vi "Dashboard Main.vi"() -> ()   [LabVIEW 2014]
uses:
  <vilib>/event_ctls.llb/eventvkey.ctl
  <vilib>/Rock Robotics/WPI/Dashboard/WPI_DashboardLogging Global.vi
  <vilib>/Utility/config.llb/Write Key (String).vi
  <vilib>/Utility/config.llb/Write Key (I32).vi
  <vilib>/Utility/config.llb/NI_LVConfig.lvlib
panel:
  in  "TCP":refnum<k5>
  in  "Rec Mode":enum32{"Stop", "Record", "Playback"}(radio)
  in  "Vision":u16(ring) items=["Camera Off", "USB Camera SW", "USB Camera HW", "IP Camera"]
  out "Camera IP":string
  out "Image Message":string="Timeout in Camera Communications"
  in  "Dashboard Tab":T1(tab)
  in  "Camera Settings":T2={"Frame Rate"=30, "Compression"=30, "Size"=1} {"Frame Rate" scale=1.0..30.0; "Size" items=["640x480", "320x240", "160x120"]}
  out "MotorChart R":cluster{"Numeric":dbl, "Numeric":dbl}(graph)
  out "MotorChart L":T3(graph)
  out "MotorSliders R":cluster{"MotorSlide1":dbl, "MotorSlide2":dbl} {"MotorSlide2" scale=-1.0..1.0 scale format="%#_2e"; "MotorSlide1" scale=-1.0..1.0 scale format="%#_2e"}
  out "MotorSliders L":T4 {"MotorSlide4 2" scale=0.0..14.0 scale format="%#_2e"; "MotorSlide2" scale=-1.0..1.0 scale format="%#_2e"; "MotorSlide1" scale=-1.0..1.0 scale format="%#_2e"}
  out "JS1 Z":dbl(slide) scale=-1.0..1.0 scale format="%#_2e"
  out "JS1 Graph":cluster{"X":dbl, "Y":dbl}[](graph)
  out "JS1 Buttons":T5
  out "JS2 Z":dbl(slide) scale=-1.0..1.0 scale format="%#_2e"
  out "JS2 Graph":cluster{"X":dbl, "Y":dbl}[](graph)
  out "JS2 Buttons":T5
  out "Mode":T6(ring)=enum."Auto Disabled"
  in  "DB Camera Config":bool
  out "fps":dbl format="%#.1g"
  out "Mbps":dbl format="%#.1g"
  out "Mbps 2":bool
  in  "DB/String 9":string
  in  "DB/String 8":string
  in  "DB/String 7":string
  in  "DB/String 6":string
  in  "DB/String 5":string
  in  "DB/String 4":string
  in  "DB/String 3":string
  in  "DB/String 2":string
  in  "DB/String 1":string
  in  "DB/String 0":string
  in  "DB/Slider 0":dbl(slide) scale=0.0..5.0
  in  "DB/Slider 1":dbl(slide) scale=0.0..5.0
  in  "DB/Slider 2":dbl(slide) scale=0.0..5.0
  in  "DB/Slider 3":dbl(slide) scale=0.0..5.0
  out "DB/LED 3":bool
  out "DB/LED 2":bool
  out "DB/LED 1":bool
  out "DB/LED 0":bool
  in  "DB/Button 3":bool
  in  "DB/Button 2":bool
  in  "DB/Button 1":bool
  in  "DB/Button 0":bool caption="New Name"
  out "FWE2":dbl
  out "Pincher Dist":dbl
  out "FWE1":dbl
  in  "FW Offset":dbl min=-1.0 max=1.0 step=0.01
  out "Fly Wheel Speed":dbl
  out "Up/Down Speed":dbl
  in  "Boolean 2":bool
  in  "Test Slider":dbl(slide) scale=0.0..100.0 scale format="%#_3g"
  in  "On/Off":bool caption="Solenoid"
  in  "Test Name":u16(ring) items=["Select the test to run...", "Example Test", "-------------------------------", "List of tests is built in robot code.", "Replace with your own automated tests."]
  in  "Test Tree":string(tree)
  in  "Motor":cluster{"Value":dbl, "Enable":bool} {"Value" scale=-1.0..1.0 scale format="%#_3g"}
  out "Progress":T7 {"Test Progress" scale=0.0..100.0}
  in  "Rev/Fwd":cluster{"Forward":bool, "Reverse":bool}
  in  "Test Ring":u16(ring) items=["Monochrome", "Color"]
  in  "Listbox":i32(listbox)
  out "Tree":string(tree)
  out "Camera Image":T8(plugin-control)
  out "Boolean":bool
  # "Left"
  # "Front"
  # "Right"
  # "Battery"
  # "This tab is a great place for autonomous settings and robot-specific values.\nPlace controls and indicators inside this tab and match name to\nDashboard Variables on robot. You can also delete this comment."
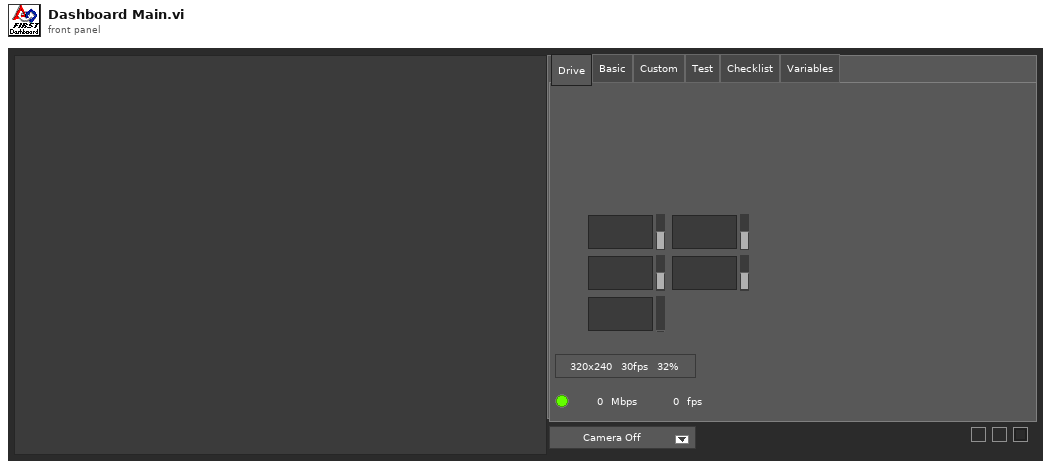
[diagram p1: front panel]
types:
  T1 = enum32{"Drive", "Basic", "Custom", "Test", "Checklist", "Variables"}
  T2 = cluster{"Frame Rate":i32, "Compression":i32, "Size":u16}
  T3 = cluster{"Numeric":dbl, "Numeric":dbl, "Battery V":dbl}
  T4 = cluster{"MotorSlide1":dbl, "MotorSlide2":dbl, "MotorSlide4 2":dbl}
  T5 = cluster{bool, bool, bool, bool, bool, bool, bool, bool, bool, bool, bool, bool}
  T6 = enum8{"Tele-Op Disabled", "Tele-Op Enabled", "Auto Disabled", "Auto Enabled", "Test Disabled", "Test Enabled", "Disconnected", "No Code", "E-Stop"}
  T7 = cluster{"Test Progress":u8, "Test Progress Text":string}
  T8 = typedef "IMAQ Image.ctl" = refnum<image>
  T9 = typedef "Image Type" = u32
  T10 = cluster{"Camera Image":refnum<vi>, "Dashboard Tab":refnum<vi>, "Boolean":refnum<vi>, "Vision":refnum<vi>, "Rec Mode":refnum<vi>, "Test Slider":refnum<vi>, "On/Off ":refnum<vi>, "Test Ring":refnum<vi>, "Rev/Fwd":refnum<vi>, "Test Name":refnum<vi>, "Motor":refnum<vi>, "Progress":refnum<vi>, "CheckList":refnum<vi>, "Tree":refnum<vi>, "Test Tree":refnum<vi>}
  T11 = cluster{"Error Strings":string, "Disable Counts":cluster{u16, u16}, "Rail Faults":cluster{u16, u16, u16}, "Robot IP":string, "DB Mode":u8, "Event Info":cluster{"Name":string, "Type":u8, "Number":u16, "Replay":u8}, "Camera Addr":string}
  T12 = cluster{"Storage":cluster{"Disk Free":u64, "RAM Block":u32, "RAM free":u32}, "CPU Utilization":cluster{"CPU % ISR":sgl, "CPU % Time Crit":sgl, "CPU % Timed Str":sgl, "CPU % High":sgl, "CPU % Above":sgl, "CPU % Normal":sgl, "CPU % Low":sgl}, "CAN":cluster{"% Bus Utilization":sgl, "Bus Off Cnt":u32, "TX_FIFO Full Cnt":u32, "Receive Error Cnt":u8, "Transmit Error Cnt":u8}, "HID":cluster{"HID Outputs":u32, "Rumble Low":u16, "Rumble High":u16}[]}
  T13 = cluster{"Status bits":cluster{"Test Mode":bool, "Autonomous":bool, "Enabled":bool, "Code Start":bool, "Brownout":bool, "Reserved 2":bool, "Reserved 3":bool, "E-Stop":bool}, "Code Trace":cluster{"Disabled":bool, "TeleOp":bool, "Auto":bool, "Test":bool}, "Controller Type":enum16{"unknown", "cRIO", "roboRio"}, "Code?":enum16{"unknown", "noCode", "code"}, "Battery V":dbl}
  T14 = cluster{"Control Bits":cluster{"TestMode":bool, "Autonomous":bool, "Enabled":bool, "FMS Present":bool, bool, bool, bool, "E-Stop":bool}, "Team Station ":u8, "Countdown":sgl, "Joystick Values":cluster{"Axes":dbl[], "Buttons":bool[], "POVs":i16[]}[]}
  T15 = cluster{"Axes":dbl[], "Buttons":bool[], "POVs":i16[]}[]
  T16 = cluster{"Axes":dbl[], "Buttons":bool[], "POVs":i16[]}
  T17 = cluster{"Buttons[0]":bool, "Buttons[1]":bool, "Buttons[2]":bool, "Buttons[3]":bool, "Buttons[4]":bool, "Buttons[5]":bool, "Buttons[6]":bool, "Buttons[7]":bool, "Buttons[8]":bool, "Buttons[9]":bool, "Buttons[10]":bool, "Buttons[11]":bool}
  T18 = typedef "NI_LVConfig.lvlib/Config Data RefNum.ctl" = refnum<k1>
  T19 = cluster{"Operation":enum16{"Update", "Clear"}, "Color Box":u32}[]
  T20 = typedef "eventvkey.ctl" = enum16{"ASCII", "Enter", "Return", "Shift", "Ctrl", "Alt", "Cmd", "Opt", "Caps", "NumLock", "Clear", "Break", "Up", "Down", "Left", "Right", "Insert", "Delete", "Home", "End", "PageUp", "PageDown", "Escape", "Help", "Pause", "ScrollLock", "F1", "F2", "F3", "F4", "F5", "F6", "F7", "F8", "F9", "F10", "F11", "F12", "F13", "F14", "F15", "F16", "F17", "F18", "F19", "F20", "F21", "F22", "F23", "F24", "Play", "VolumeUp", "VolumeDown", "Mute", "Two Byte Char"}
  T21 = cluster{"Image Size":bool, "Image Type":bool, "Pixel Value":bool, "ROI Information":bool, "Zoom Factor":bool}
  T22 = enum8{"Enabled", "Disabled", "Disabled and Grayed Out"}
  T23 = cluster{"Operation":enum16{"Update", "Clear"}, "Color Box":u32}
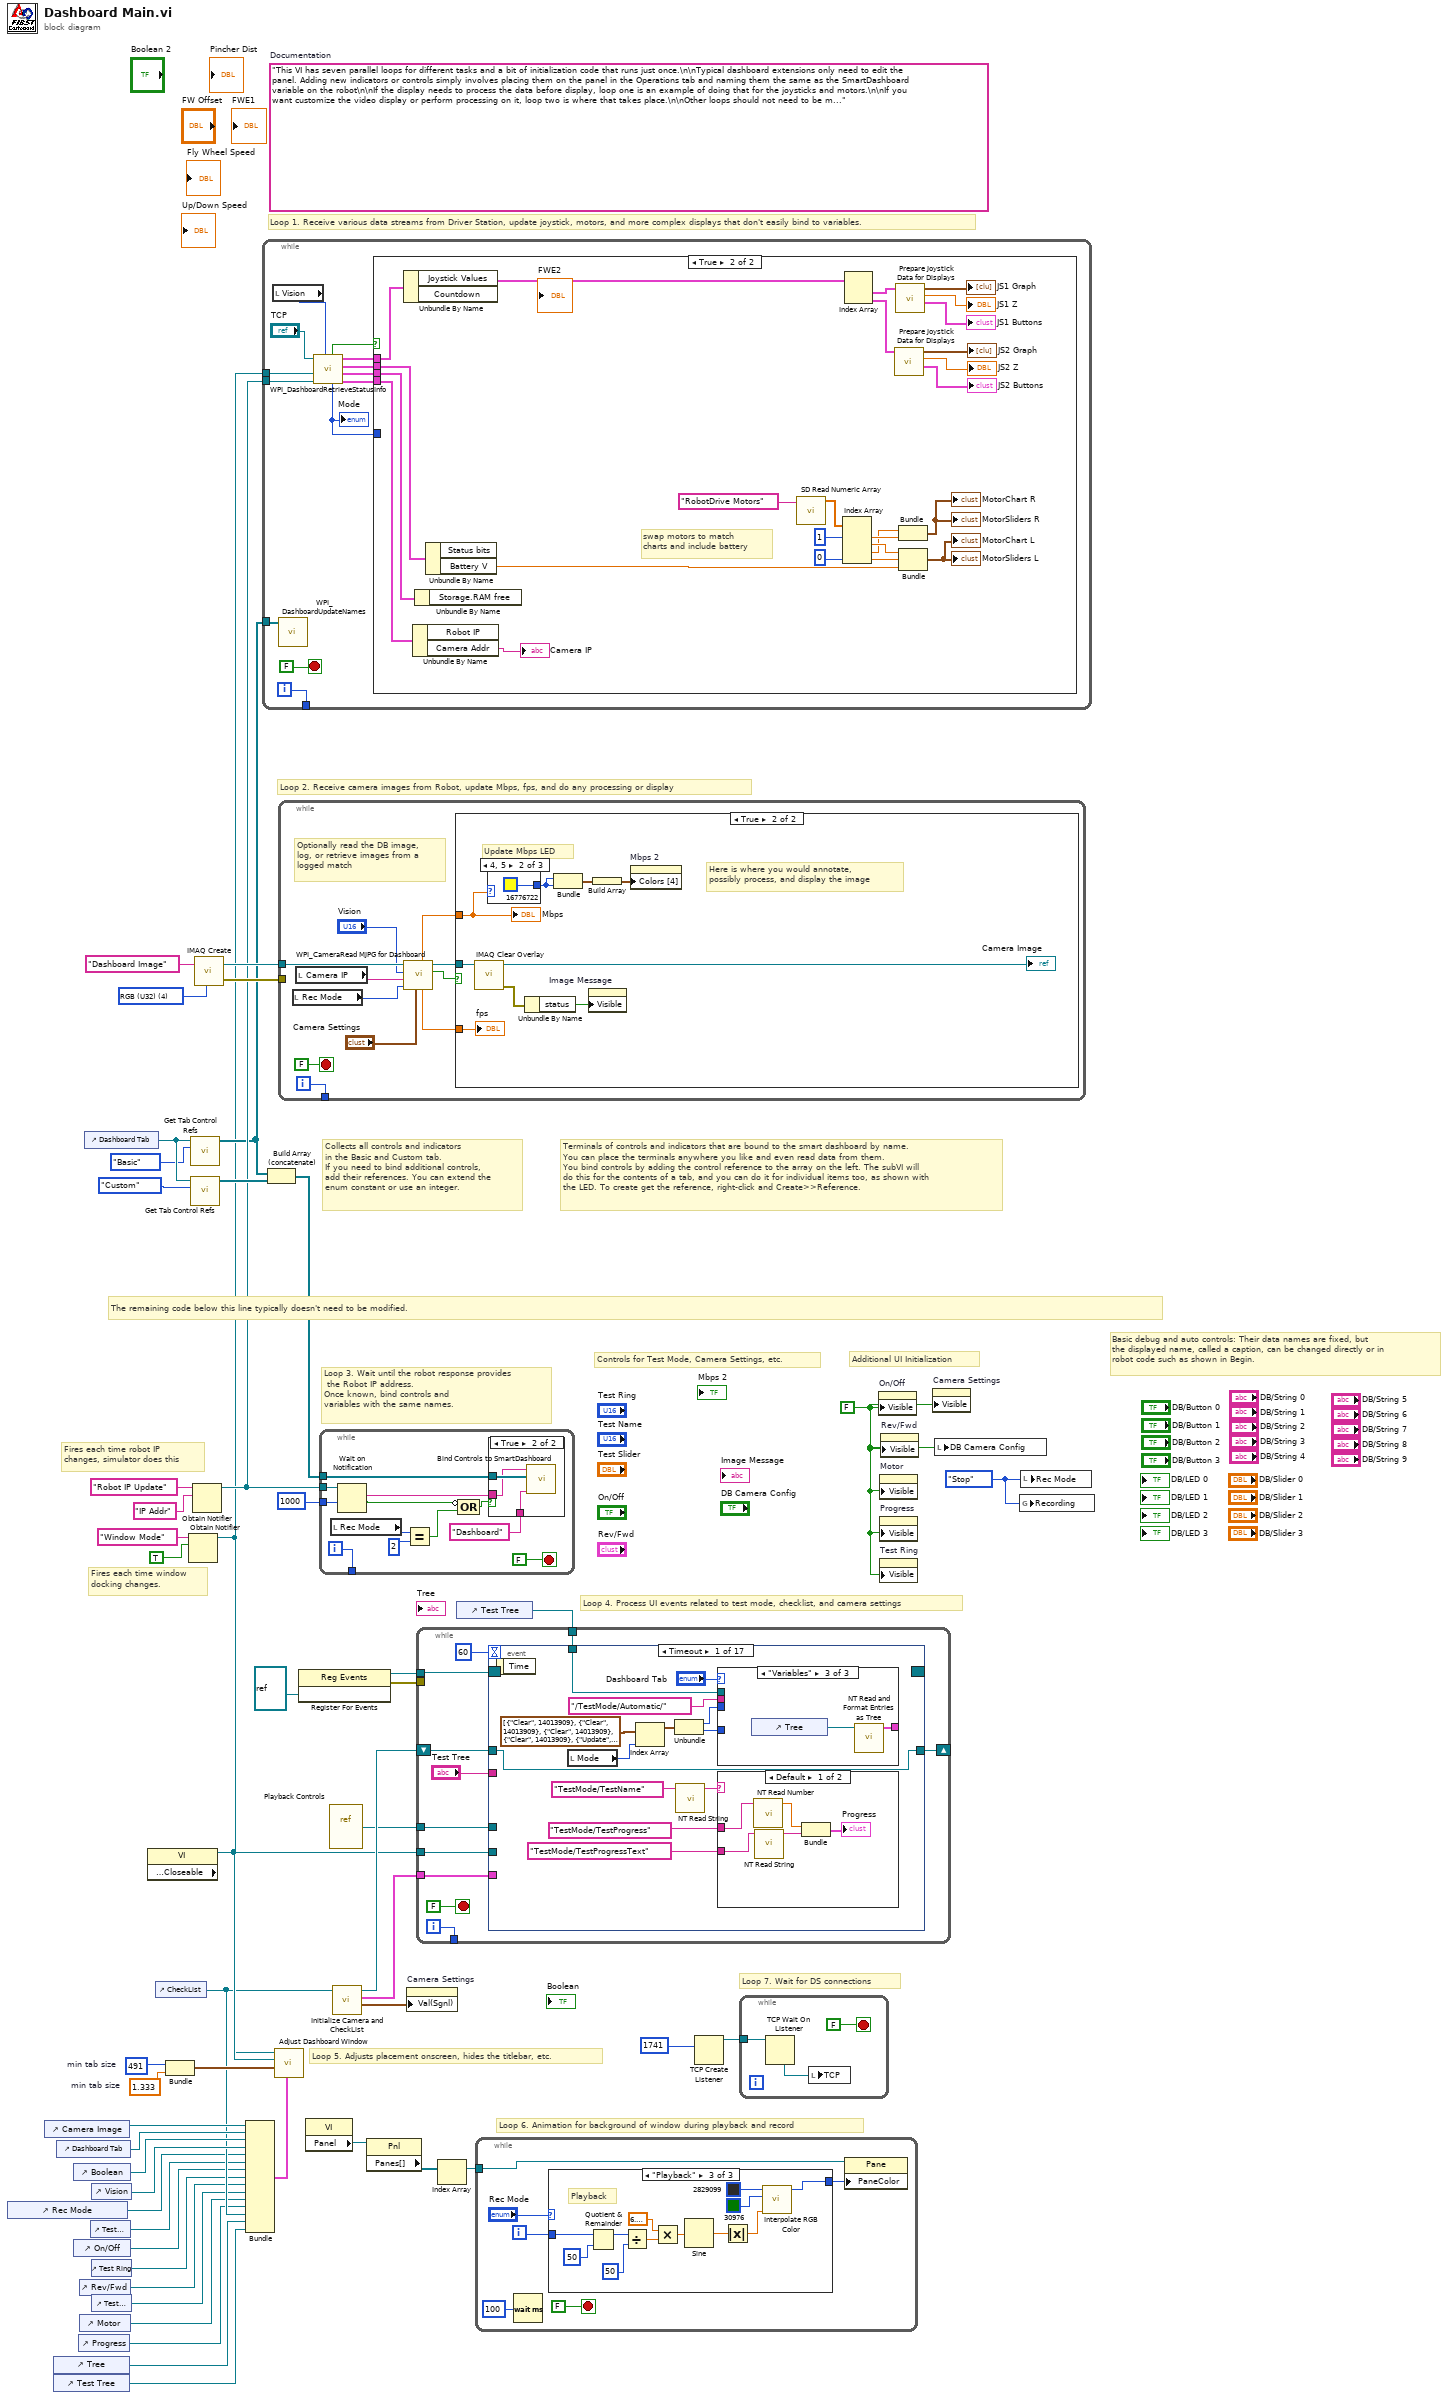
[diagram p0: block diagram]
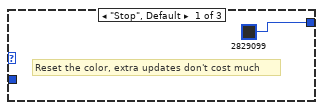
[diagram p3: hidden frame]
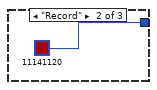
[diagram p4: hidden frame]
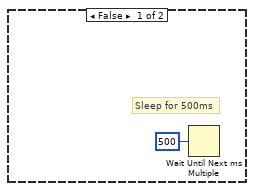
[diagram p6: hidden frame]
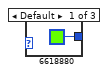
[diagram p7: hidden frame]
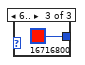
[diagram p8: hidden frame]
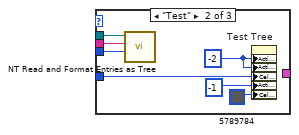
[diagram p10: hidden frame]
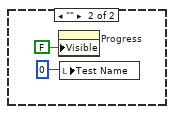
[diagram p11: hidden frame]
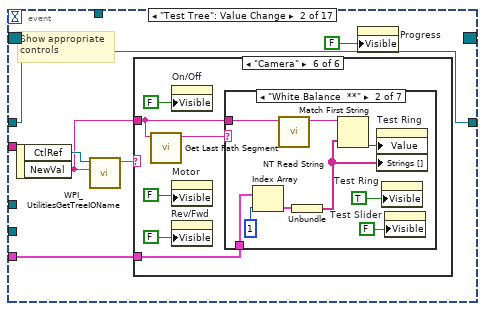
[diagram p12: hidden frame]
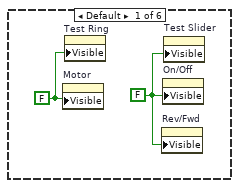
[diagram p13: hidden frame]
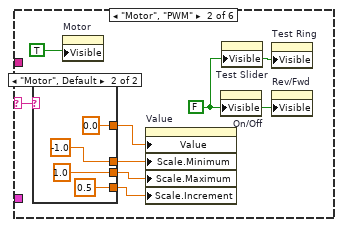
[diagram p14: hidden frame]
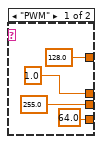
[diagram p15: hidden frame]
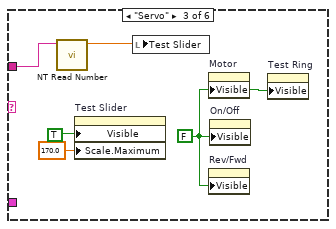
[diagram p16: hidden frame]
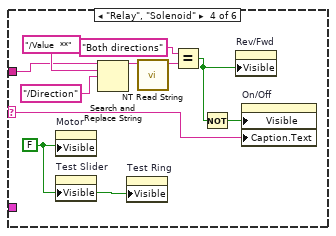
[diagram p17: hidden frame]
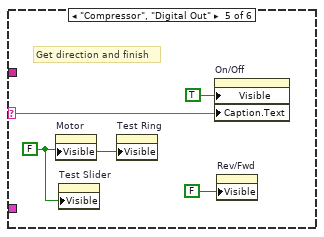
[diagram p18: hidden frame]
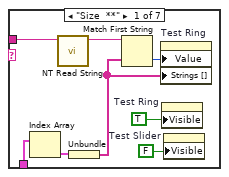
[diagram p19: hidden frame]
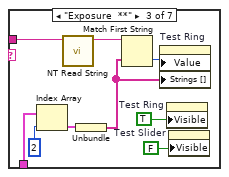
[diagram p20: hidden frame]
diagram:
  w24 = 491  # min tab size
  w23 = 1.333  # min tab size
  w32 = enum32{"Stop", "Record", "Playback"}."Stop" ("Rec Mode")
  w6 = FALSE ("Visible")
  (unwired) "This VI has seven parallel loops for different tasks and a bit of initialization code that runs just once.\n\nTypical dashboard extensions only need to edit the panel. Adding new indicators or controls simply involves placing them on the panel in the Operations tab and naming them the same as the SmartDashboard variable on the robot\n\nIf the display needs to process the data before display, loop one is an example of doing that for the joysticks and motors.\n\nIf you want customize the video display or perform processing on it, loop two is where that takes place.\n\nOther loops should not need to be modified. They are pretty standard, and document the task they perform."  # Documentation
  w52 = T9 4 items=["Grayscale (U8)", "Grayscale (I16)", "Grayscale (SGL)", "Complex (CSG)", "RGB (U32)", "HSL (U32)", "RGB (U64)"] ("Image Type")
  # "Loop 7. Wait for DS connections"
  # "Basic debug and auto controls: Their data names are fixed, but\nthe displayed name, called a caption, can be changed directly or in\nrobot code such as shown in Begin."
  # "Controls for Test Mode, Camera Settings, etc."
  # "Additional UI Initialization"
  # "Loop 6. Animation for background of window during playback and record"
  # "Fires each time robot IP\nchanges, simulator does this"
  # "Fires each time window\ndocking changes."
  # "Collects all controls and indicators\nin the Basic and Custom tab.\nIf you need to bind additional controls,\nadd their references. You can extend the\nenum constant or use an integer."
  # "The remaining code below this line typically doesn't need to be modified."
  # "Loop 4. Process UI events related to test mode, checklist, and camera settings"
  # "Terminals of controls and indicators that are bound to the smart dashboard by name.\nYou can place the terminals anywhere you like and even read data from them.\nYou bind controls by adding the control reference to the array on the left. The subVI will\ndo this for the contents of a tab, and you can do it for individual items too, as shown with\nthe LED. To create get the reference, right-click and Create>>Reference."
  # "Loop 3. Wait until the robot response provides\n the Robot IP address.\nOnce known, bind controls and\nvariables with the same names."
  # "Loop 5. Adjusts placement onscreen, hides the titlebar, etc."
  # "Loop 1. Receive various data streams from Driver Station, update joystick, motors, and more complex displays that don't easily bind to variables."
  # "Loop 2. Receive camera images from Robot, update Mbps, fps, and do any processing or display"
  n1 = control-ref of="Rec Mode"() -> (w12:refnum<vi>)
  n2 = control-ref of="Camera Image"() -> (w27:refnum<vi>)
  n3 = control-ref of="Tree"() -> (w16:refnum<vi>)
  n4 = control-ref of="Test Tree"() -> (w15:refnum<vi>)
  n5 = control-ref of="Dashboard Tab"() -> (w26:refnum<vi>)
  n6 = control-ref of="Boolean"() -> (w21:refnum<vi>)
  n7 = control-ref of="On/Off"() -> (w10:refnum<vi>)
  n8 = control-ref of="Progress"() -> (w7:refnum<vi>)
  n9 = control-ref of="Rev/Fwd"() -> (w8:refnum<vi>)
  n10 = control-ref of="Motor"() -> (w13:refnum<vi>)
  n11 = control-ref of="Dashboard Tab"() -> (w30:refnum<vi>)
  n12 = control-ref of="Test Slider"() -> (w11:refnum<vi>)
  n13 = control-ref of="Vision"() -> (w25:refnum<vi>)
  n14 = control-ref of="Test Ring"() -> (w9:refnum<vi>)
  n15 = control-ref of="Test Name"() -> (w14:refnum<vi>)
  n16 = property class="VI" props=["Front Panel.Closeable"]() -> (reference out=w31:refnum<vi>)  [unwired: 2 in, 2 out]
  n17 = control-ref of="CheckList"() -> (w17:refnum<vi>)
  n18 = Bundle("min tab size"=w24, "min tab size"=w23) -> (w22:cluster{"min tab size":i32, "min tab size":dbl})  [unwired: 1 in]
  n19 = Obtain Notifier(name (unnamed)="Window Mode", notification data type=TRUE) -> (notifier out=w3:refnum<notifier>)  [unwired: 2 in, 2 out]
  n20 = call <vilib>:"Get Tab Control Refs.vi"("Page Index"=T1."Basic" ("Dashboard Tab"), "TabControl in"=w30) -> ("ControlsOnPage"=w4:refnum<vi>[])  [unwired: 9 in]
  n21 = call <vilib>:"Get Tab Control Refs.vi"("Page Index"=T1."Custom" ("Dashboard Tab"), "TabControl in"=w30) -> ("ControlsOnPage"=w29:refnum<vi>[])  [unwired: 9 in]
  n22 = Obtain Notifier(name (unnamed)="Robot IP Update", notification data type="IP Addr" ("name (unnamed)")) -> (notifier out=w5:refnum<notifier>)  [unwired: 2 in, 2 out]
  n23 = call "IMAQ Create"("Image Name"="Dashboard Image", "Image Type"=w52) -> ("New Image"=w50:T8, "error out"=w49:errorcluster)  [unwired: 2 in, 1 out]
  n24 = Bundle("Camera Image"=w27, "Dashboard Tab"=w26, "Boolean"=w21, "Vision"=w25, "Rec Mode"=w12, "Test Slider"=w11, "On/Off"=w10, "Test Ring"=w9, "Rev/Fwd"=w8, "Test Name"=w14, "Motor"=w13, "Progress"=w7, "CheckList"=w17, "Tree"=w16, "Test Tree"=w15) -> (w18:T10)  [unwired: 1 in]
  n25 = while {
    tunnel: [w64] -> _
    tunnel: w5 -> [w58]
    tunnel: w4 -> [w57]
    tunnel: w3 -> [w53]
    i -> [w64]
    stop <- FALSE stop-if-true
    n26 = local read "Vision"() -> (w55:u16)
    n27 = call <vilib>:"WPI_DashboardUpdateNames.vi"("Controls on Tab"=w57) -> ()  [unwired: 11 in]
    n28 = call <vilib>:"WPI_DashboardRetrieveStatusInfo.vi"("Vision"=w55, "Binding Refnum"=w58, "Window Mode Notifier"=w53, "TCP Cnx"="TCP") -> ("Power and Errors"=w59:T11, "Robot Metrics"=w62:T12, "Status Info"=w63:T13, "Control Info"=w60:T14, "Robot Mode"=w56:T6, "Process?"=w61:bool)  [unwired: 2 in]
    "Mode" <- w56
    n29 = case shown="True" w61 {
      tunnel: w63 -> [_ w90]
      tunnel: w62 -> [_ w89]
      tunnel: w60 -> [_ w88]
      tunnel: w59 -> [_ w87]
      tunnel: w56 -> [_ _]
      frame False {
      }
      frame True {
        # "swap motors to match\ncharts and include battery"
        n30 = Unbundle By Name(w88) -> ("Joystick Values"=w75:T15)  [unwired: 1 out]
        n31 = Unbundle By Name(w87) -> ("Camera Addr"=→"Camera IP":string)  [unwired: 1 out]
        n32 = Unbundle By Name(w89) -> ()  [unwired: 1 out]
        n33 = Unbundle By Name(w90) -> ("Battery V"=w76:dbl)  [unwired: 1 out]
        n34 = call <vilib>:"SD Read Numeric Array.vi"("Name"="RobotDrive Motors") -> ("Numeric Array"=w78:dbl[])  [unwired: 8 in, 2 out]
        n35 = Index Array(array=w78, index #1=1, index #4=0) -> (element #1=w82:dbl, element #2=w83:dbl, element #3=w81:dbl, element #4=w86:dbl)  [unwired: 2 in]
        n36 = Index Array(array=w75) -> (element #1=w74:T16, element #2=w69:T16)  [unwired: 2 in]
        n37 = call "Prepare Joystick Data for Displays.vi"("Joystick Values"=w69) -> ("Buttons"=→"JS2 Buttons":T17, "Z Axis"=→"JS2 Z":dbl, "Cartesian Data"=→"JS2 Graph":cluster{"X axis":dbl, "X axis":dbl}[])  [unwired: 8 in]
        n38 = call "Prepare Joystick Data for Displays.vi"("Joystick Values"=w74) -> ("Buttons"=→"JS1 Buttons":T17, "Z Axis"=→"JS1 Z":dbl, "Cartesian Data"=→"JS1 Graph":cluster{"X axis":dbl, "X axis":dbl}[])  [unwired: 8 in]
        n39 = Bundle("Numeric"=w81, "Numeric"=w82) -> (→"MotorChart R" →"MotorSliders R":cluster{"Numeric":dbl, "Numeric":dbl})  [unwired: 1 in]
        n40 = Bundle("Numeric"=w83, "Numeric"=w86, "Battery V"=w76) -> (→"MotorChart L" →"MotorSliders L":T3)  [unwired: 1 in]
      }
    }
  }
  n41 = Build Array (concatenate)(w4, w29) -> (w28:refnum<vi>[])
  n42 = call "Adjust Dashboard Window.vi"("Sizing Refnums"=w18, "Size Constraints"=w22, "VI"=w31, "Notifier in"=w3) -> ()  [unwired: 8 in]
  n43 = while {
    tunnel: w50 -> [w99]
    tunnel: w49 -> [_]
    tunnel: [w100] -> _
    i -> [w100]
    stop <- FALSE stop-if-true
    # "Optionally read the DB image,\nlog, or retrieve images from a\nlogged match"
    n44 = local read "Rec Mode"() -> (w93:enum32{"Stop", "Record", "Playback"})
    n45 = local read "Camera IP"() -> (w91:string)
    n46 = call <vilib>:"WPI_CameraRead MJPG for Dashboard.vi"("Camera Settings"="Camera Settings", "Rec Mode"=w93, "Camera IP"=w91, "Camera Mode"="Vision", "Refnum in"=w99) -> ("Active"=w97:bool, "Refnum out"=w98:T8, "FPS"=w96:dbl, "Bandwidth (Mbps)"=w95:dbl)  [unwired: 3 in]
    n47 = case shown="True" w97 {
      tunnel: w98 -> [_ w106]
      tunnel: w95 -> [_ w105]
      tunnel: w96 -> [_ w103]
      frame False {
        # "Sleep for 500ms"
        n48 = Wait Until Next ms Multiple(millisecond multiple=u32 500) -> ()  [unwired: 1 out]
      }
      frame True {
        # "Here is where you would annotate,\npossibly process, and display the image"
        # "Update Mbps LED"
        n49 = call "IMAQ Clear Overlay"("Image"=w106) -> ("error out"=w110:errorcluster, "Image Out"=→"Camera Image":T8)  [unwired: 2 in, 7 out]
        n50 = case shown="4, 5" w105 {
          tunnel: [u32 6618880 ("Color Box") u32 16776722 ("Color Box") u32 16716800 ("Color Box")] -> w107
          frame Default {
          }
          frame 4, 5 {
          }
          frame 6.. {
          }
        }
        n51 = Unbundle By Name(w110) -> ("status"=w111:bool)
        n52 = Bundle("Color Box"=w107, "Color Box"=w107) -> (w109:cluster{"Color Box":u32, "Color Box":u32})  [unwired: 1 out]
        n53 = property on="Image Message" class="Str"("Visible"=w111) -> ()  [unwired: 2 in, 2 out]
        n54 = Build Array(w109) -> (w108:cluster{"Color Box":u32, "Color Box":u32}[])
        n55 = property on="Mbps 2" class="Bool (strict)"("Colors [4]"=w108) -> ()  [unwired: 2 in, 2 out]
        "Mbps" <- w105
        "fps" <- w103
      }
    }
  }
  n56 = register-events(refnum<vi> refnum) -> (reference out=w36:refnum<event-registration>, error out=w35:errorcluster)  [unwired: 2 in]
  n57 = property class="VI"() -> ("Panel"=w39:refnum<vi>)  [unwired: 2 in, 2 out]
  n58 = while {
    tunnel: w28 -> [w126]
    tunnel: w5 -> [w124]
    tunnel: [w122] -> _
    tunnel: u32 1000 ("milliseconds to wait") -> [w121]
    i -> [w122]
    stop <- FALSE stop-if-true
    n59 = local read "Rec Mode"() -> (w117:enum32{"Stop", "Record", "Playback"})
    n60 = Wait on Notification(notifier=w124, timeout in ms (-1)=w121) -> (notification=w123:string, timed out?=w119:bool)  [unwired: 2 in, 2 out]
    n61 = Equal?(x=w117, y=u16 2 ("Rec Mode")) -> (x = y?=w118:bool)
    n62 = Compound Arithmetic op=OR(invert w119, w118) -> (w120:bool)
    n63 = case shown="True" w120 {
      tunnel: w126 -> [_ w129]
      tunnel: w123 -> [_ w128]
      tunnel: "Dashboard" -> [_ w127]
      frame False {
      }
      frame True {
        n64 = call <vilib>:"Bind Controls to SmartDashboard.vi"("Client Name"=w127, "Bound Control Refs"=w129, "Server IP Address"=w128) -> ()  [unwired: 9 in]
      }
    }
  }
  n65 = vi-ref "Playback Controls.vi"() -> (w37:refnum<vi>)
  n66 = call "Initialize Camera and CheckList.vi"("ListBox in"=w17) -> ("Cluster"=w43:cluster{"value":i32, "value":i32, "index":i32}, "Array"=w44:cluster{string[]}[], "File Refnum"=w42:T18)  [unwired: 8 in]
  n67 = property class="Pnl"(reference=w39) -> ("Panes[]"=w40:refnum<vi>[])  [unwired: 1 in, 2 out]
  n68 = property on="Camera Settings" class="Clust (strict)"("Val(Sgnl)"=w43) -> ()  [unwired: 2 in, 2 out]
  n69 = Index Array(array=w40) -> (element=w38:refnum<vi>)  [unwired: 1 in]
  n70 = control-ref of="Test Tree"() -> (w41:refnum<vi>)
  n71 = while {
    tunnel: w44 -> [w137]
    shift-right: [w136] -> _
    shift-left: w42 -> [w135]
    tunnel: [w134] -> _
    tunnel: w41 -> [w133]
    tunnel: w37 -> [w132]
    tunnel: w36 -> [w131]
    tunnel: w35 -> [_]
    tunnel: w31 -> [w130]
    i -> [w134]
    stop <- FALSE stop-if-true
    n72 = event shown="[0] Timeout" {
      selector: w131 -> [_ _ _ _ _ _ _ _ _ _ _ _ _ _ _ _ _]
      dyn-events: [_ _ _ _ _ _ _ _ _ _ _ _ _ w375 _ _ _] -> _
      timeout: u32 60 ("milliseconds to wait") -> [_ _ _ _ _ _ _ _ _ _ _ _ _ _ _ _ _]
      tunnel: w133 -> [w149 _ _ _ _ _ _ _ _ _ _ _ _ _ _ _ _]
      tunnel: "Test Tree" -> [_ _ _ _ _ _ _ _ w344 w352 w354 w358 w366 _ _ _ _]
      tunnel: w137 -> [_ w171 _ _ _ _ w308 w338 _ _ _ _ _ _ _ _ _]
      tunnel: [w145 w170 w269 w274 w282 w294 w307 w331 w343 w350 w353 w357 w365 w377 w391 w392 w402] -> w136
      tunnel: w135 -> [w145 w170 w269 w274 w282 w294 w306 w331 w343 w350 w353 w357 w365 w377 w391 w392 w402]
      tunnel: w132 -> [_ _ _ _ _ _ _ _ _ _ _ _ _ w378 _ w395 _]
      tunnel: w130 -> [_ _ _ _ _ _ _ _ _ _ _ _ _ w373 _ _ _]
      event Timeout {
        n73 = event-data() -> ()  [unwired: 1 in, 1 out]
        n74 = local read "Mode"() -> (w148:T6)
        n75 = Index Array(array=T19 [{"Operation"=enum."Clear", "Color Box"=14013909}, {"Operation"=enum."Clear", "Color Box"=14013909}, {"Operation"=enum."Clear", "Color Box"=14013909}, {"Operation"=enum."Clear", "Color Box"=14013909}, {"Operation"=enum."Update", "Color Box"=14013909}, {"Operation"=enum."Update", "Color Box"=16777215}, {"Operation"=enum."Clear", "Color Box"=14013909}, {"Operation"=enum."Clear", "Color Box"=14013909}, {"Operation"=enum."Clear", "Color Box"=14013909}], index=w148) -> (element=w143:T23)
        n76 = Unbundle(w143) -> ("Operation"=w142:enum16{"Update", "Clear"}, "Color Box"=w141:u32)
        n77 = call <vilib>:"NT Read String.vi"("Name"="TestMode/TestName") -> ("String"=w152:string)  [unwired: 9 in, 1 out]
        n78 = case shown="\"Variables\"" "Dashboard Tab" {
          tunnel: w149 -> [_ w160 _]
          tunnel: "/TestMode/Automatic/" ("Name Pattern") -> [_ w159 _]
          tunnel: w142 -> [_ w158 _]
          tunnel: [_ _ w162] -> _
          tunnel: w141 -> [_ w154 _]
          frame "Custom", Default {
          }
          frame "Test" {
            w157 = -2 ("Active Item:Row Number")
            n79 = call <vilib>:"NT Read and Format Entries as Tree.vi"("Operation"=w158, "Name Pattern"=w159, "Tree Refnum"=w160) -> ()  [unwired: 7 in, 2 out]
            n80 = property on="Test Tree" class="Tree (strict)"("Active Item Row Number"=w157, "ActiveColNum"=w157, "CellBG"=w154, "Active Item Row Number"=-1 ("Active Item:Row Number"), "CellBG"=u32 5789784 ("Color Box")) -> ()  [unwired: 2 in, 2 out]
          }
          frame "Variables" {
            n81 = control-ref of="Tree"() -> (w161:refnum<vi>)
            n82 = call <vilib>:"NT Read and Format Entries as Tree.vi"("Tree Refnum"=w161) -> ("Formatted Strings"=w162:cluster{"Name":string, "Value":string}[])  [unwired: 9 in, 1 out]
          }
        }
        n83 = case shown="Default" w152 {
          tunnel: "TestMode/TestProgress" ("Name") -> [w164 _]
          tunnel: "TestMode/TestProgressText" ("Name") -> [w163 _]
          frame Default {
            n84 = call <vilib>:"NT Read Number.vi"("Name"=w164) -> ("Numeric"=w165:dbl)  [unwired: 9 in, 1 out]
            n85 = call <vilib>:"NT Read String.vi"("Name"=w163) -> ("String"=w166:string)  [unwired: 9 in, 1 out]
            n86 = Bundle("Numeric"=w165, "String"=w166) -> (→"Progress":cluster{"Numeric":dbl, "String":string})  [unwired: 1 in]
          }
          frame "" {
            n87 = property on="Progress" class="Clust (strict)"("Visible"=FALSE) -> ()  [unwired: 2 in, 2 out]
            n88 = local write "Test Name"(u16 0) -> ()
          }
        }
      }
      event "Test Tree": Value Change {
        # "Show appropriate\ncontrols"
        n89 = event-data() -> ("CtlRef"=w174:refnum<vi>, "NewVal"=w172:string)  [unwired: 1 in]
        n90 = call <vilib>:"WPI_UtilitiesGetTreeIOName.vi"("NewVal"=w172, "TreeControl in"=w174) -> ("I/O Name"=w175:string)  [unwired: 9 in]
        n91 = case shown="\"Camera\"" w175 {
          selector: w175 -> [_ w182 _ w200 w209 _]
          tunnel: w172 -> [_ _ w197 w199 _ w216]
          tunnel: w171 -> [_ _ _ _ _ w215]
          frame Default {
            w177 = FALSE ("Visible")
            w176 = FALSE ("Visible")
            n92 = property on="Motor" class="Clust (strict)"("Visible"=w176) -> ()  [unwired: 2 in, 2 out]
            n93 = property on="Test Ring" class="Ring (strict)"("Visible"=w176) -> ()  [unwired: 2 in, 2 out]
            n94 = property on="Rev/Fwd" class="Clust (strict)"("Visible"=w177) -> ()  [unwired: 2 in, 2 out]
            n95 = property on="On/Off" class="Bool (strict)"("Visible"=w177) -> ()  [unwired: 2 in, 2 out]
            n96 = property on="Test Slider" class="Slide (strict)"("Visible"=w177) -> ()  [unwired: 2 in, 2 out]
          }
          frame "Motor", "PWM" {
            w183 = FALSE ("Visible")
            n97 = case shown="\"Motor\", Default" w182 {
              tunnel: [1.0 ("Value") -1.0 ("Value")] -> w181
              tunnel: [255.0 ("Value") 1.0 ("Value")] -> w180
              tunnel: [128.0 ("Value") 0.0 ("Value")] -> w179
              tunnel: [64.0 ("Value") 0.5 ("Value")] -> w178
              frame "PWM" {
              }
              frame "Motor", Default {
              }
            }
            n98 = property on="Motor" class="Clust (strict)"("Visible"=TRUE) -> ()  [unwired: 2 in, 2 out]
            n99 = property on="Value" class="Slide (strict)"("Value"=w179, "Scale.Minimum"=w181, "Scale.Maximum"=w180, "Scale.Increment"=w178) -> ()  [unwired: 2 in, 2 out]
            n100 = property on="On/Off" class="Bool (strict)"("Visible"=w183) -> ()  [unwired: 2 in, 2 out]
            n101 = property on="Test Slider" class="Slide (strict)"("Visible"=w183) -> ()  [unwired: 2 in, 2 out]
            n102 = property on="Test Ring" class="Ring (strict)"("Visible"=w183) -> ()  [unwired: 2 in, 2 out]
            n103 = property on="Rev/Fwd" class="Clust (strict)"("Visible"=w183) -> ()  [unwired: 2 in, 2 out]
          }
          frame "Servo" {
            w195 = FALSE ("Visible")
            n104 = call <vilib>:"NT Read Number.vi"("Name"=w197) -> ("Numeric"=w196:dbl)  [unwired: 9 in, 1 out]
            n105 = property on="Test Slider" class="Slide (strict)"("Visible"=TRUE, "Scale.Maximum"=170.0 ("Scale.Range:Maximum")) -> ()  [unwired: 2 in, 2 out]
            n106 = local write "Test Slider"(w196) -> ()
            n107 = property on="Motor" class="Clust (strict)"("Visible"=w195) -> ()  [unwired: 2 in, 2 out]
            n108 = property on="Rev/Fwd" class="Clust (strict)"("Visible"=w195) -> ()  [unwired: 2 in, 2 out]
            n109 = property on="On/Off" class="Bool (strict)"("Visible"=w195) -> ()  [unwired: 2 in, 2 out]
            n110 = property on="Test Ring" class="Ring (strict)"("Visible"=w195) -> ()  [unwired: 2 in, 2 out]
          }
          frame "Relay", "Solenoid" {
            w198 = FALSE ("Visible")
            n111 = property on="Motor" class="Clust (strict)"("Visible"=w198) -> ()  [unwired: 2 in, 2 out]
            n112 = property on="Test Slider" class="Slide (strict)"("Visible"=w198) -> ()  [unwired: 2 in, 2 out]
            n113 = Search and Replace String(input string=w199, search string="/Value  **", replace string="/Direction") -> (result string=w205:string)  [unwired: 5 in, 3 out]
            n114 = property on="Test Ring" class="Ring (strict)"("Visible"=w198) -> ()  [unwired: 2 in, 2 out]
            n115 = call <vilib>:"NT Read String.vi"("Name"=w205) -> ("String"=w203:string)  [unwired: 9 in, 1 out]
            n116 = Equal?(x="Both directions", y=w203) -> (x = y?=w201:bool)
            n117 = Not(x=w201) -> (.not. x?=w202:bool)
            n118 = property on="Rev/Fwd" class="Clust (strict)"("Visible"=w201) -> ()  [unwired: 2 in, 2 out]
            n119 = property on="On/Off" class="Bool (strict)"("Visible"=w202, "Caption.Text"=w200) -> ()  [unwired: 2 in, 2 out]
          }
          frame "Compressor", "Digital Out" {
            w208 = FALSE ("Visible")
            # "Get direction and finish"
            n120 = property on="Motor" class="Clust (strict)"("Visible"=w208) -> ()  [unwired: 2 in, 2 out]
            n121 = property on="Test Slider" class="Slide (strict)"("Visible"=w208) -> ()  [unwired: 2 in, 2 out]
            n122 = property on="Test Ring" class="Ring (strict)"("Visible"=w208) -> ()  [unwired: 2 in, 2 out]
            n123 = property on="On/Off" class="Bool (strict)"("Visible"=TRUE, "Caption.Text"=w209) -> ()  [unwired: 2 in, 2 out]
            n124 = property on="Rev/Fwd" class="Clust (strict)"("Visible"=FALSE) -> ()  [unwired: 2 in, 2 out]
          }
          frame "Camera" {
            n125 = call <vilib>:"Get Last Path Segment.vi"("String in"=w216) -> ("String out"=w217:string)  [unwired: 10 in]
            n126 = property on="On/Off" class="Bool (strict)"("Visible"=FALSE) -> ()  [unwired: 2 in, 2 out]
            n127 = property on="Motor" class="Clust (strict)"("Visible"=FALSE) -> ()  [unwired: 2 in, 2 out]
            n128 = property on="Rev/Fwd" class="Clust (strict)"("Visible"=FALSE) -> ()  [unwired: 2 in, 2 out]
            n129 = case shown="\"White Balance  **\"" w217 {
              tunnel: w216 -> [w223 w232 w241 w250 w259 _ w265]
              tunnel: w215 -> [w221 w229 w238 w247 w256 _ _]
              frame "Size  **" {
                n130 = Index Array(array=w221) -> (element=w220:cluster{string[]})  [unwired: 1 in]
                n131 = call <vilib>:"NT Read String.vi"("Name"=w223) -> ("String"=w222:string)  [unwired: 9 in, 1 out]
                n132 = Unbundle(w220) -> (w218:string[])
                n133 = Match First String(2:w218, 3:w222) -> (0:w219:i32)  [unwired: 1 out]
                n134 = property on="Test Ring" class="Ring (strict)"("Value"=w219, "Strings []"=w218) -> ()  [unwired: 2 in, 2 out]
                n135 = property on="Test Ring" class="Ring (strict)"("Visible"=TRUE) -> ()  [unwired: 2 in, 2 out]
                n136 = property on="Test Slider" class="Slide (strict)"("Visible"=FALSE) -> ()  [unwired: 2 in, 2 out]
              }
              frame "White Balance  **" {
                n137 = Index Array(array=w229, index=1) -> (element=w230:cluster{string[]})
                n138 = call <vilib>:"NT Read String.vi"("Name"=w232) -> ("String"=w231:string)  [unwired: 9 in, 1 out]
                n139 = Unbundle(w230) -> (w227:string[])
                n140 = Match First String(2:w227, 3:w231) -> (0:w226:i32)  [unwired: 1 out]
                n141 = property on="Test Ring" class="Ring (strict)"("Value"=w226, "Strings []"=w227) -> ()  [unwired: 2 in, 2 out]
                n142 = property on="Test Ring" class="Ring (strict)"("Visible"=TRUE) -> ()  [unwired: 2 in, 2 out]
                n143 = property on="Test Slider" class="Slide (strict)"("Visible"=FALSE) -> ()  [unwired: 2 in, 2 out]
              }
              frame "Exposure  **" {
                n144 = Index Array(array=w238, index=2) -> (element=w239:cluster{string[]})
                n145 = call <vilib>:"NT Read String.vi"("Name"=w241) -> ("String"=w240:string)  [unwired: 9 in, 1 out]
                n146 = Unbundle(w239) -> (w235:string[])
                n147 = Match First String(2:w235, 3:w240) -> (0:w236:i32)  [unwired: 1 out]
                n148 = property on="Test Ring" class="Ring (strict)"("Value"=w236, "Strings []"=w235) -> ()  [unwired: 2 in, 2 out]
                n149 = property on="Test Ring" class="Ring (strict)"("Visible"=TRUE) -> ()  [unwired: 2 in, 2 out]
                n150 = property on="Test Slider" class="Slide (strict)"("Visible"=FALSE) -> ()  [unwired: 2 in, 2 out]
              }
              frame "Exposure Priority  **" {
                n151 = Index Array(array=w247, index=3) -> (element=w248:cluster{string[]})
                n152 = call <vilib>:"NT Read String.vi"("Name"=w250) -> ("String"=w249:string)  [unwired: 9 in, 1 out]
                n153 = Unbundle(w248) -> (w244:string[])
                n154 = Match First String(2:w244, 3:w249) -> (0:w245:i32)  [unwired: 1 out]
                n155 = property on="Test Ring" class="Ring (strict)"("Value"=w245, "Strings []"=w244) -> ()  [unwired: 2 in, 2 out]
                n156 = property on="Test Ring" class="Ring (strict)"("Visible"=TRUE) -> ()  [unwired: 2 in, 2 out]
                n157 = property on="Test Slider" class="Slide (strict)"("Visible"=FALSE) -> ()  [unwired: 2 in, 2 out]
              }
              frame "Color Enable  **" {
                n158 = Index Array(array=w256, index=4) -> (element=w257:cluster{string[]})
                n159 = call <vilib>:"NT Read String.vi"("Name"=w259) -> ("String"=w258:string)  [unwired: 9 in, 1 out]
                n160 = Unbundle(w257) -> (w253:string[])
                n161 = Match First String(2:w253, 3:w258) -> (0:w254:i32)  [unwired: 1 out]
                n162 = property on="Test Ring" class="Ring (strict)"("Value"=w254, "Strings []"=w253) -> ()  [unwired: 2 in, 2 out]
                n163 = property on="Test Ring" class="Ring (strict)"("Visible"=TRUE) -> ()  [unwired: 2 in, 2 out]
                n164 = property on="Test Slider" class="Slide (strict)"("Visible"=FALSE) -> ()  [unwired: 2 in, 2 out]
              }
              frame Default {
                n165 = property on="Test Ring" class="Ring (strict)"("Visible"=FALSE) -> ()  [unwired: 2 in, 2 out]
                n166 = property on="Test Slider" class="Slide (strict)"("Visible"=FALSE) -> ()  [unwired: 2 in, 2 out]
              }
              frame "Brightness  **", "Color Level  **", "Compression  **", "FPS  **", "Sharpness  **" {
                n167 = call <vilib>:"NT Read Number.vi"("Name"=w265) -> ("Numeric"=w264:dbl)  [unwired: 9 in, 1 out]
                n168 = local write "Test Slider"(w264) -> ()
                n169 = property on="Test Slider" class="Slide (strict)"("Visible"=TRUE, "Scale.Maximum"=100.0 ("Scale.Range:Maximum")) -> ()  [unwired: 2 in, 2 out]
                n170 = property on="Test Ring" class="Ring (strict)"("Visible"=FALSE) -> ()  [unwired: 2 in, 2 out]
              }
            }
          }
        }
        n171 = property on="Progress" class="Clust (strict)"("Visible"=FALSE) -> ()  [unwired: 2 in, 2 out]
      }
      event "Test Name": Mouse Enter {
        # "Populate the ring with the list of tests"
        n172 = event-data() -> ()  [unwired: 1 in, 1 out]
        n173 = call <vilib>:"NT Read String Array.vi"("Name"="TestMode/TestList") -> ("String Array"=w273:string[])  [unwired: 9 in, 1 out]
        n174 = Build Array (concatenate)("Select the test to run...", w273) -> (w272:string[])
        n175 = property on="Test Name" class="Ring (strict)"("Strings []"=w272) -> ()  [unwired: 2 in, 2 out]
      }
      event "Test Name": Value Change {
        w275 = FALSE ("Visible")
        # "Tell the robot the test name to run"
        n176 = event-data() -> ("NewVal"=w279:u16)  [unwired: 1 in]
        n177 = property on="Test Name" class="Ring (strict)"() -> ("Strings []"=w280:string[])  [unwired: 2 in, 2 out]
        n178 = local write "Progress"(T7 {"Test Progress"=0, "Test Progress Text"=""} ("Progress")) -> ()
        n179 = Index Array(array=w280, index=w279) -> (element=w278:string)
        n180 = call <vilib>:"NT Write String.vi"("String"=w278, "Name"="TestMode/TestName") -> ()  [unwired: 9 in, 1 out]
        n181 = property on="Progress" class="Clust (strict)"("Visible"=TRUE) -> ()  [unwired: 2 in, 2 out]
        n182 = property on="Motor" class="Clust (strict)"("Visible"=w275) -> ()  [unwired: 2 in, 2 out]
        n183 = property on="Test Slider" class="Slide (strict)"("Visible"=w275) -> ()  [unwired: 2 in, 2 out]
        n184 = property on="On/Off" class="Bool (strict)"("Visible"=w275) -> ()  [unwired: 2 in, 2 out]
        n185 = property on="Rev/Fwd" class="Clust (strict)"("Visible"=w275) -> ()  [unwired: 2 in, 2 out]
        n186 = property on="Test Ring" class="Ring (strict)"("Visible"=w275) -> ()  [unwired: 2 in, 2 out]
      }
      event "Listbox": Double Click {
        # "Shift clears all"
        # "Update symbols on the listbox"
        n187 = event-data() -> ("PlatMods.Shift"=w283:bool, "Row"=w285:i32)  [unwired: 1 in]
        n188 = case shown="True" w283 {
          tunnel: w285 -> [w289 _]
          tunnel: 1 -> [w288 _]
          frame False {
            n189 = property on="Listbox" class="LstBox (strict)"() -> ("Item Symbols"=w287:i32[])  [unwired: 2 in, 2 out]
            n190 = Replace Array Subset(array=w287, new element=w288, index=w289) -> (w286:i32[])
            n191 = property on="Listbox" class="LstBox (strict)"("Item Symbols"=w286) -> ()  [unwired: 2 in, 2 out]
          }
          frame True {
            w290 = 0 ("Top Row")
            n192 = property on="Listbox" class="LstBox (strict)"() -> ("Number of Rows"=w292:u32)  [unwired: 2 in, 2 out]
            n193 = Initialize Array(0, w292) -> (w291:i32[])
            n194 = property on="Listbox" class="LstBox (strict)"("Top Row"=w290, "Value"=w290, "Item Symbols"=w291) -> ()  [unwired: 2 in, 2 out]
          }
        }
      }
      event "Listbox": Key Down {
        # "Update symbols on the listbox\nLeft and right keys check and uncheck"
        n195 = event-data() -> ("VKey"=w296:T20)  [unwired: 1 in]
        n196 = case shown="\"Left\", \"Right\"" w296 {
          selector: w296 -> [w301 _]
          tunnel: eventvkey."Left" ("VKey") -> [w299 _]
          frame "Left", "Right" {
            n197 = Equal?(x=w299, y=w301) -> (x = y?=w300:bool)
            n198 = Select(t=0, s=w300, f=1) -> (s? t:f=w302:i32)
            n199 = property on="Listbox" class="LstBox (strict)"() -> ("Item Symbols"=w305:i32[])  [unwired: 2 in, 2 out]
            n200 = Replace Array Subset(array=w305, new element=w302, index="Listbox") -> (w304:i32[])
            n201 = property on="Listbox" class="LstBox (strict)"("Item Symbols"=w304) -> ()  [unwired: 2 in, 2 out]
          }
          frame Default {
          }
        }
      }
      event "DB Camera Config": Value Change {
        # "Show or hide the cluster of controls, store in ini file"
        n202 = event-data() -> ("NewVal"=w309:bool)  [unwired: 1 in]
        n203 = case shown="False" w309 {
          tunnel: w308 -> [w318 _]
          tunnel: [w311 w329] -> w307
          tunnel: w306 -> [w310 w329]
          frame False {
            w325 = "Camera"
            w328 = FALSE ("Visible")
            n204 = local read "Camera Settings"() -> (w317:T2)
            n205 = Index Array(array=w318) -> (element=w321:cluster{string[]})  [unwired: 1 in]
            n206 = Unbundle(w317) -> ("Frame Rate"=w316:i32, "Compression"=w315:i32, "Size"=w319:u16)
            n207 = Unbundle(w321) -> (w320:string[])
            n208 = Index Array(array=w320, index=w319) -> (element=w314:string)
            n209 = call-poly <vilib>:"Write Key.vi"("section"=w325, "value"=w314, "key"="Size", "refnum"=w310) -> ("refnum out"=w327:T18)  [unwired: 2 in, 5 out]
            n210 = call-poly <vilib>:"Write Key.vi"("section"=w325, "value"=w316, "key"="FrameRate", "refnum"=w327) -> ("refnum out"=w326:T18)  [unwired: 1 in, 6 out]
            n211 = property on="Camera Settings" class="Clust (strict)"("Visible"=w328) -> ()  [unwired: 2 in, 2 out]
            n212 = local write "DB Camera Config"(w328) -> ()
            n213 = call-poly <vilib>:"Write Key.vi"("section"=w325, "value"=w315, "key"="Compression", "refnum"=w326) -> ("refnum out"=w312:T18)  [unwired: 1 in, 6 out]
            n214 = call <vilib>:"Close Config Data.vi"("refnum"=w312) -> ("file path"=w313:path)  [unwired: 2 in, 8 out]
            n215 = call <vilib>:"Open Config Data.vi"("configuration file path"=w313) -> ("refnum"=w311:T18)  [unwired: 8 in, 2 out]
          }
          frame True {
            n216 = property on="Camera Settings" class="Clust (strict)"("Visible"=TRUE) -> ()  [unwired: 2 in, 2 out]
          }
        }
      }
      event "Camera Settings": Value Change {
        # "Update summary string when any elements of DB camera change"
        n217 = event-data() -> ("NewVal"=w342:T2)  [unwired: 1 in]
        n218 = Index Array(array=w338) -> (element=w337:cluster{string[]})  [unwired: 1 in]
        n219 = Unbundle(w342) -> ("Frame Rate"=w333:i32, "Compression"=w332:i32, "Size"=w335:u16)
        n220 = Unbundle(w337) -> (w336:string[])
        n221 = Index Array(array=w336, index=w335) -> (element=w334:string)
        n222 = Format Into String(format string="%s   %dfps   %d%%", w334, w333, w332) -> (resulting string=w339:string)  [unwired: 2 in, 1 out]
        n223 = Build Array(w339) -> (w340:string[])
        n224 = property on="DB Camera Config" class="Bool (strict)"("Strings [4]"=w340) -> ()  [unwired: 2 in, 2 out]
      }
      event "Motor.Enable": Value Change {
        # "When the test mode otor enable helper is set, update that\ntree row item's value"
        n225 = event-data() -> ("NewVal"=w348:bool)  [unwired: 1 in]
        n226 = Unbundle("Motor") -> ("Value"=w347:dbl)  [unwired: 1 out]
        n227 = Select(t=w347, s=w348, f=0.0) -> (s? t:f=w345:dbl)
        n228 = call <vilib>:"NT Write Number.vi"("Numeric"=w345, "Name"=w344) -> ()  [unwired: 9 in, 1 out]
      }
      event "Test Slider": Value Change {
        # "When the test mode slider helper is set, update that\ntree row item's value"
        n229 = event-data() -> ("NewVal"=w351:dbl)  [unwired: 1 in]
        n230 = call <vilib>:"NT Write Number.vi"("Numeric"=w351, "Name"=w352) -> ()  [unwired: 9 in, 1 out]
      }
      event "On/Off": Value Change {
        # "When the test mode on/off helper value is set, update that\ntree row item's value"
        n231 = event-data() -> ("NewVal"=w356:bool)  [unwired: 1 in]
        n232 = Boolean To (0,1)(Boolean=w356) -> (0, 1=w355:i16)
        n233 = call <vilib>:"NT Write Number.vi"("Numeric"=w355, "Name"=w354) -> ()  [unwired: 9 in, 1 out]
      }
      event "Rev/Fwd": Value Change {
        # "When the test mode helper value for relays is set, update that\ntree row item's value"
        n234 = event-data() -> ("NewVal.Forward"=w364:bool, "NewVal.Reverse"=w363:bool)  [unwired: 1 in]
        n235 = Boolean To (0,1)(Boolean=w364) -> (0, 1=w360:i16)
        n236 = Boolean To (0,1)(Boolean=w363) -> (0, 1=w362:i16)
        n237 = Negate(x=w362) -> (-x=w361:i16)
        n238 = Add(x=w360, y=w361) -> (x+y=w359:i16)
        n239 = call <vilib>:"NT Write Number.vi"("Numeric"=w359, "Name"=w358) -> ()  [unwired: 9 in, 1 out]
      }
      event "Test Ring": Value Change {
        # "When a test mode helper value is selected from the ring,\nset the tree item's variable to the string value"
        n240 = event-data() -> ("NewVal"=w368:u16)  [unwired: 1 in]
        n241 = property on="Test Ring" class="Ring (strict)"() -> ("Strings []"=w369:string[])  [unwired: 2 in, 2 out]
        n242 = Index Array(array=w369, index=w368) -> (element=w367:string)
        n243 = call <vilib>:"NT Write String.vi"("String"=w367, "Name"=w366) -> ()  [unwired: 9 in, 1 out]
      }
      event "Rec Mode": Value Change {
        # "Update globals for recording mode and path to read log from.\nClear when logging and let NetworkTables set path for vision to\nuse."
        n244 = event-data() -> ("NewVal"=w379:enum32{"Stop", "Record", "Playback"})  [unwired: 1 in]
        n245 = global write "WPI_DashboardLogging Global.vi" "Logging Filename"(path "") -> ()
        n246 = case shown="\"Playback\"" w379 {
          tunnel: w378 -> [_ w381 w389]
          tunnel: [_ _ w388] -> w375
          tunnel: [_ _ w387] -> _
          tunnel: w373 -> [_ _ w385]
          tunnel: cluster{i32, i32} {-250, 170} -> [_ _ w384]
          tunnel: [_ _ T21 {"Image Size"=TRUE, "Image Type"=TRUE, "Pixel Value"=TRUE, "ROI Information"=TRUE, "Zoom Factor"=FALSE} ("Image Information Shown:All Elements")] -> w371
          tunnel: [_ _ TRUE ("Zoom Factor")] -> w370
          frame Default {
          }
          frame "Stop", "Record" {
            # "Place Window too"
            n247 = invoke class="VI" method="FP.Close"(reference=w381) -> (reference out=w380:refnum<vi>)  [unwired: 2 in, 2 out]
            n248 = invoke class="VI" method="Abort VI"(reference=w380) -> ()  [unwired: 2 in, 3 out]
          }
          frame "Playback" {
            n249 = call "Open Playback Panel.vi"("Offset"=w384, "DB VI Ref"=w385, "Playback in"=w389) -> ("Playback out"=w386:refnum<vi>)  [unwired: 8 in]
            n250 = register-events(w386) -> (reference out=w388:refnum<event-registration>, error out=w387:errorcluster)  [unwired: 2 in]
          }
        }
        n251 = global write "WPI_DashboardLogging Global.vi" "Recording"(w379) -> ()
        n252 = property on="Camera Image" class="ImageControl"("Image Information Shown"=w371, "Image Information Visible"=w370) -> ()  [unwired: 2 in, 2 out]
        n253 = call <vilib>:"WPI_DashboardNT Log FieldName Cache.vi"("Operation"=enum16{"Lookup/Add", "Index", "Clear"}."Clear") -> ()  [unwired: 8 in, 3 out]
      }
      event Panel Close {
        w390 = enum32{"Stop", "Record", "Playback"}."Stop" ("Rec Mode")
        # "Playback window has been closed, abort"
        n254 = event-data() -> ()  [unwired: 1 in, 4 out]
        n255 = local write "Rec Mode"(w390) -> ()
        n256 = global write "WPI_DashboardLogging Global.vi" "Recording"(w390) -> ()
      }
      event Panel Close {
        # "Abort playback window and ourself"
        n257 = event-data() -> ()  [unwired: 1 in, 4 out]
        n258 = invoke class="VI" method="FP.Close"(reference=w395) -> (reference out=w394:refnum<vi>)  [unwired: 2 in, 2 out]
        n259 = invoke class="VI" method="Abort VI"(reference=w394) -> (error out=w393:errorcluster)  [unwired: 2 in, 2 out]
        n260 = invoke class="VI" method="Abort VI"(error in=w393) -> ()  [unwired: 2 in, 3 out]
      }
      event "Vision": Value Change {
        # "Enable/Disable Compression slider.\nHW USB is hard-coded into the camera"
        n261 = event-data() -> ("NewVal"=w401:u16)  [unwired: 1 in]
        n262 = Equal?(x=w401, y=u32 2 ("milliseconds to wait")) -> (x = y?=w399:bool)
        n263 = Select(t=T22."Disabled and Grayed Out" ("Disabled"), s=w399, f=T22."Enabled" ("Disabled")) -> (s? t:f=w396:T22)
        n264 = property on="Compression" class="Slide (strict)"("DisabledEnum"=w396) -> ()  [unwired: 2 in, 2 out]
      }
    }
  }
  n265 = while {
    tunnel: w38 -> [w404]
    i -> [w407]
    stop <- FALSE stop-if-true
    n266 = Wait (ms)(milliseconds to wait=u32 100) -> ()  [unwired: 1 out]
    n267 = case shown="\"Playback\"" "Rec Mode" {
      tunnel: w407 -> [_ _ w422]
      tunnel: [u32 2829099 ("Base Color") u32 11141120 ("Target Color") w411] -> w403
      frame "Stop", Default {
        # "Reset the color, extra updates don't cost much"
      }
      frame "Record" {
      }
      frame "Playback" {
        # "Playback"
        n268 = Quotient & Remainder(x=w422, y=u32 50 ("milliseconds to wait")) -> (x-y*floor(x/y)=w418:u32)  [unwired: 1 out]
        n269 = Divide(x=w418, y=u32 50 ("milliseconds to wait")) -> (x/y=w415:dbl)
        n270 = Multiply(x=6.283185307179586, y=w415) -> (x*y=w420:dbl)
        n271 = Sine(x=w420) -> (sin(x)=w419:dbl)
        n272 = Absolute Value(x=w419) -> (abs(x)=w412:dbl)
        n273 = call "Interpolate RGB Color.vi"("Proportion"=w412, "Target Color"=u32 30976, "Base Color"=u32 2829099) -> ("Result Color"=w411:u32)  [unwired: 8 in]
      }
    }
    n274 = property class="Pane"(reference=w404, "PaneColor"=w403) -> ()  [unwired: 1 in, 2 out]
  }
  n275 = TCP Create Listener(10:u16 1741 ("timeout ms (25000)")) -> (3:w1:refnum<k5>)  [unwired: 4 in, 2 out]
  n276 = while {
    tunnel: w1 -> [w424]
    stop <- FALSE stop-if-true
    n277 = TCP Wait On Listener(11:w424) -> (4:w423:refnum<k5>)  [unwired: 3 in, 4 out]
    n278 = local write "TCP"(w423) -> ()
  }
  n279 = property on="On/Off" class="Bool (strict)"("Visible"=w6) -> ()  [unwired: 2 in, 2 out]
  n280 = property on="Motor" class="Clust (strict)"("Visible"=w6) -> ()  [unwired: 2 in, 2 out]
  n281 = property on="Progress" class="Clust (strict)"("Visible"=w6) -> ()  [unwired: 2 in, 2 out]
  n282 = property on="Test Ring" class="Ring (strict)"("Visible"=w6) -> ()  [unwired: 2 in, 2 out]
  n283 = property on="Rev/Fwd" class="Clust (strict)"("Visible"=w6) -> ()  [unwired: 2 in, 2 out]
  n284 = property on="Camera Settings" class="Clust (strict)"("Visible"=w6) -> ()  [unwired: 2 in, 2 out]
  n285 = local write "DB Camera Config"(w6) -> ()
  n286 = global write "WPI_DashboardLogging Global.vi" "Recording"(w32) -> ()
  n287 = local write "Rec Mode"(w32) -> ()
